vi "SetAPSxAttribute.vi"(8 "error in (no error)":errorcluster caption="错误输入（无错误）", 9 "Param2":i32, 10 "Param1":i32, 11 "hASIC":i32) -> (0 "error out":errorcluster caption="错误输出", 1 "Message":string, 3 "hASIC out":i32)   [LabVIEW 2020]
doc: "该模板用于创建子VI。"
uses:
  APSx.dll/APSx.dll
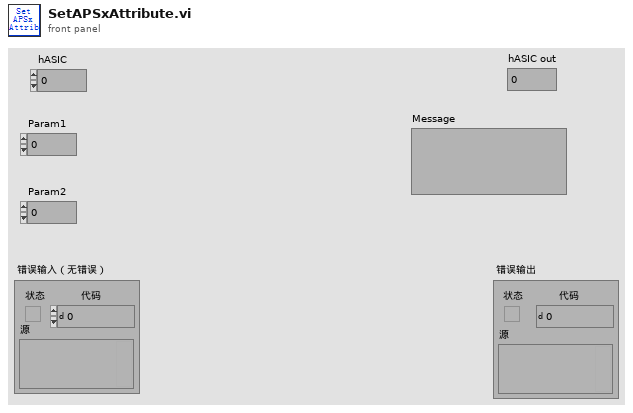
[diagram p1: front panel]
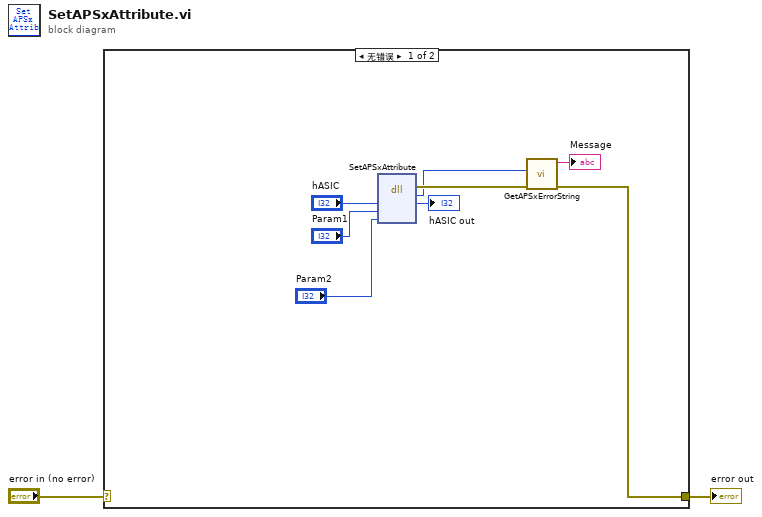
[diagram p0: block diagram]
diagram:
  n1 = case shown="无错误" "error in (no error)" {
    selector: "error in (no error)" -> [_ w11]
    tunnel: [w7 w11] -> w1
    frame No Error {
      n2 = dll-call lib="PTH2iabs CUsersFengDesktop传感器对中台传感器对中台labviewSourcesAPSx.dllAPSx.dll" fn="SetAPSxAttribute"("hASIC"="hASIC", "Param1"="Param1", "Param2"="Param2") -> (error out=w8:errorcluster, "Code"=w6:i32, "hASIC"=→"hASIC out":i32)  [unwired: 5 in, 1 out]
      n3 = call "GetAPSxErrorString.vi"("error in (no error)"=w8, "ErrorCode"=w6) -> ("error out"=w7:errorcluster, "Message"=→"Message":string)  [unwired: 8 in]
    }
    frame Error {
    }
  }
  "error out" <- w1
